vi "lib XML Parse Content.vi"(8 "error in (no error)":errorcluster, 10 "XML Line":string, 11 "XML Topic":string) -> (0 "error out":errorcluster, 2 "XML Line dup":string, 3 "Content":string)   [LabVIEW 2024]
uses:
  <vilib>/Utility/error.llb/Trim Whitespace One-Sided.vi
  <vilib>/regexp/Match Regular Expression.xnode
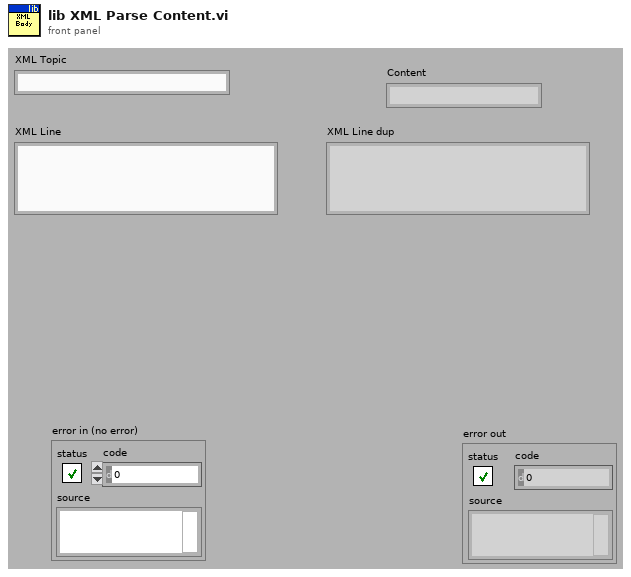
[diagram p1: front panel]
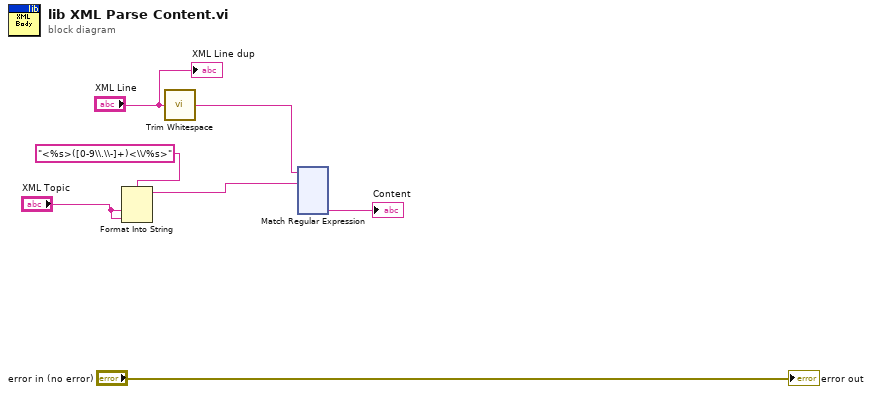
[diagram p0: block diagram]
diagram:
  n1 = Format Into String(format string="<%s>([0-9\\.\\-]+)<\\/%s>" ("regular expression"), "XML Topic", "XML Topic") -> (resulting string=w4:string)  [unwired: 2 in, 1 out]
  n2 = call <vilib>:"Trim Whitespace.vi"("string"="XML Line") -> ("trimmed string"=w6:string)  [unwired: 1 in]
  n3 = xnode "Match Regular Expression"("input string"=w6, "regular expression"=w4) -> ("submatch 1"=→"Content":string)  [unwired: 4 in, 5 out]
  "error out" <- "error in (no error)"
  "XML Line dup" <- "XML Line"
